vi "Initialize Simulated KUKA youBot.vi"(8 "error in":errorcluster, 11 "robot ID":string) -> (0 "error out":errorcluster, 3 "simulated KUKA youBot host out":refnum<class "NI_Robotics_KUKA youBot Host_Sim.lvclass">)   [LabVIEW 2017, in "NI_Robotics_KUKA youBot Host.lvlib" / "NI_Robotics_KUKA youBot Host_Sim.lvclass"]
doc: "Initializes a simulation host interface to a simulated KUKA youBot."
uses:
  <vilib>/robotics/KUKA youBot/Sim Host Interface/NI_Robotics_KUKA youBot Host_Sim.lvclass
  c:/Program Files (x86)/National Instruments/LabVIEW 2017/vi.lib/robotics/KUKA youBot/Host Interface/NI_Robotics_KUKA youBot Host Interface.lvclass
  <vilib>/robotics/KUKA youBot/Host Interface/NI_Robotics_KUKA youBot Host Interface.lvclass/NI_Robotics_KUKA youBot Host Interface.ctl
  <vilib>/robotics/KUKA youBot/Basic Device/Arm Sim/NI_Robotics_KUKA youBot Arm_Sim.lvclass
  c:/Program Files (x86)/National Instruments/LabVIEW 2017/vi.lib/robotics/KUKA youBot/Basic Device/Arm/NI_Robotics_KUKA youBot Arm.lvclass
  <vilib>/robotics/KUKA youBot/Basic Device/Mobile Platform Sim/NI_Robotics_KUKA youBot Platform_Sim.lvclass
  c:/Program Files (x86)/National Instruments/LabVIEW 2017/vi.lib/robotics/KUKA youBot/Basic Device/Mobile Platform/NI_Robotics_KUKA youBot Platform.lvclass
  <vilib>/robotics/KUKA youBot/Host Interface/NI_Robotics_KUKA youBot Host Interface.lvclass
  <vilib>/robotics/Utilities/NI_Robotics Utilities.lvlib
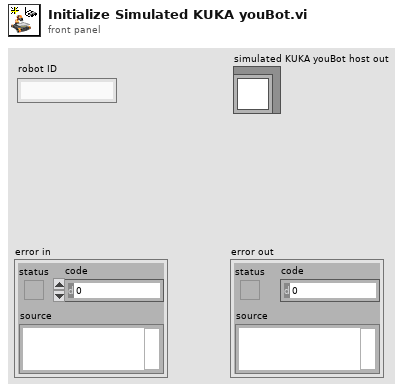
[diagram p1: front panel]
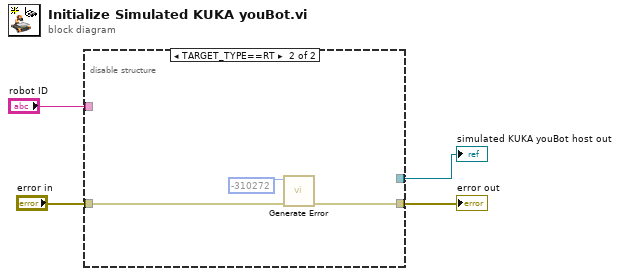
[diagram p0: block diagram]
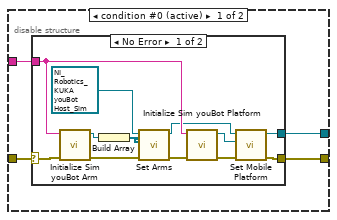
[diagram p2: hidden frame]
diagram:
  n1 = disable-structure shown="TARGET_TYPE==RT" {
    disable-tunnel: "error in" -> [w8 w22]
    disable-tunnel: "robot ID" -> [w7 _]
    disable-tunnel: [w6 _] -> w2
    disable-tunnel: [w5 w23] -> w1
    frame condition #0 (active) {
      n2 = case shown="No Error" w8 {
        selector: w8 -> [w20 w21]
        tunnel: w7 -> [w18 _]
        tunnel: [w17 _] -> w6
        tunnel: [w15 w21] -> w5
        frame No Error {
          n3 = call <vilib>:"Initialize Sim youBot Arm.vi"("error in"=w20, "Robot ID"=w18) -> ("error out"=w13:errorcluster, "NI_Robotics_KUKA youBot Arm_Sim out"=w12:refnum<class "NI_Robotics_KUKA youBot Arm_Sim.lvclass">)  [unwired: 8 in]
          n4 = Build Array(w12) -> (w11:refnum<class "NI_Robotics_KUKA youBot Arm_Sim.lvclass">[])
          n5 = call <vilib>:"Set Arms.vi"("error in (no error)"=w13, "arms"=w11, "KUKA youBot host in"=refnum<class "NI_Robotics_KUKA youBot Host_Sim.lvclass"> refnum ("NI_Robotics_KUKA youBot Host.lvlib:NI_Robotics_KUKA youBot Host_Sim.lvclass")) -> ("error out"=w14:errorcluster, "KUKA youBot host out"=w9:refnum<class "NI_Robotics_KUKA youBot Host_Sim.lvclass">)  [unwired: 7 in]
          n6 = call <vilib>:"Initialize Sim youBot Platform.vi"("error in"=w14, "robot ID"=w18) -> ("error out"=w19:errorcluster, "simulated KUKA youBot platform out"=w16:refnum<class "NI_Robotics_KUKA youBot Platform_Sim.lvclass">)  [unwired: 8 in]
          n7 = call <vilib>:"Set Mobile Platform.vi"("error in (no error)"=w19, "KUKA youBot platform in"=w16, "KUKA youBot host in"=w9) -> ("error out"=w15:errorcluster, "KUKA youBot host out"=w17:refnum<class "NI_Robotics_KUKA youBot Host_Sim.lvclass">)  [unwired: 7 in]
        }
        frame Error {
        }
      }
    }
    frame condition #1 {
      n8 = call <vilib>:"Generate Error.vi"("error in (no error)"=w22, "code"=-310272) -> ("error out"=w23:errorcluster)  [unwired: 9 in]
    }
  }
  "error out" <- w1
  "simulated KUKA youBot host out" <- w2
